vi "PLC.Dial800.OPC Read.vi"(6 "Timeout_ms":i32=500, 7 "Waif for Update":bool, 8 "error in (no error)":errorcluster, 9 "IncludeSN":bool=TRUE, 10 "Var URLs":T2[](array[typedef]), 11 "PLC Variables In":T1) -> (0 "error out":errorcluster, 1 "Duration(s)":dbl format="%.3f", 3 "PLC Variables":T1)   [LabVIEW 2018]
uses:
  PLC.Dial800.Var URL Item.ctl
  PLC.Dial800.VarNameSelector.ctl
  PLC.800 Variables.ctl
  <vilib>/KATE/Time/Time Utils.lvlib
panel:
  out "Durs":dbl[](array[numeric]) format="%.3f"
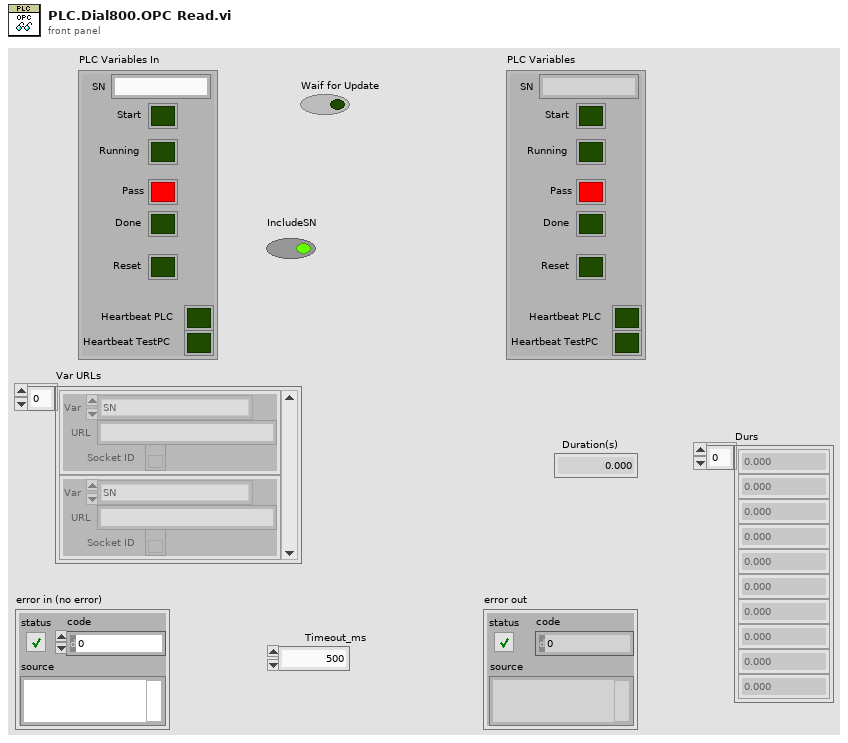
[diagram p1: front panel]
types:
  T1 = typedef "PLC.800 Variables.ctl" = cluster{"SN":string, "Start":bool, "Pass":bool, "Done":bool, "Running":bool, "Heartbeat PLC":bool, "Heartbeat TestPC":bool, "Reset":bool}
  T2 = typedef "PLC.Dial800.Var URL Item.ctl" = cluster{"Var":T3, "URL":string, "Socket ID":refnum<k13>}
  T3 = typedef "PLC.Dial800.VarNameSelector.ctl" = enum16{"SN", "Reset", "HeartBeat_PLC", "Heartbeat_PC", "Start", "Running", "Done", "Pass"}
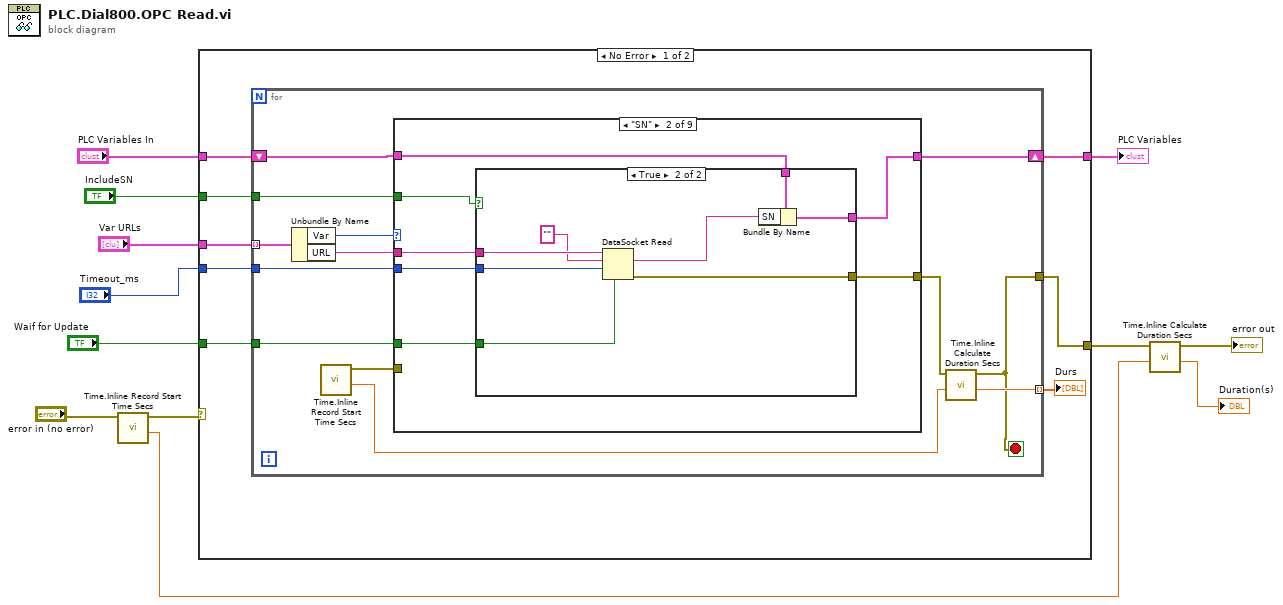
[diagram p0: block diagram]
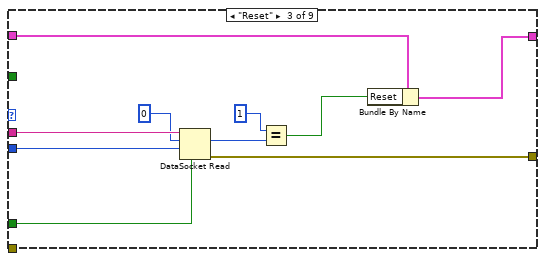
[diagram p4: hidden frame]
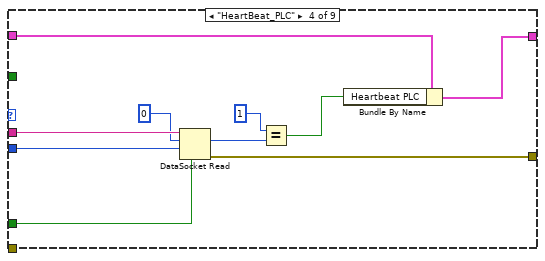
[diagram p5: hidden frame]
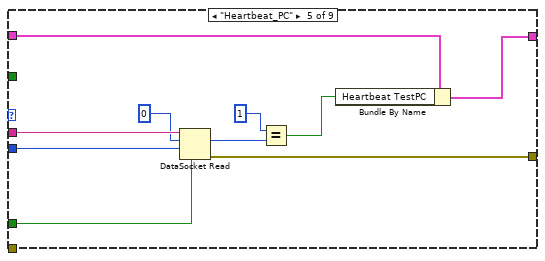
[diagram p6: hidden frame]
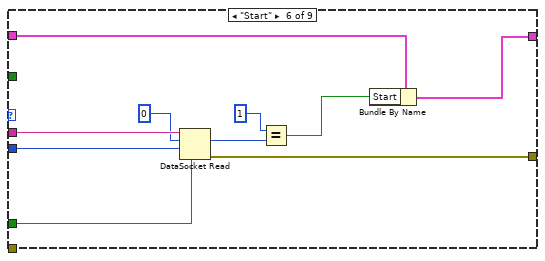
[diagram p7: hidden frame]
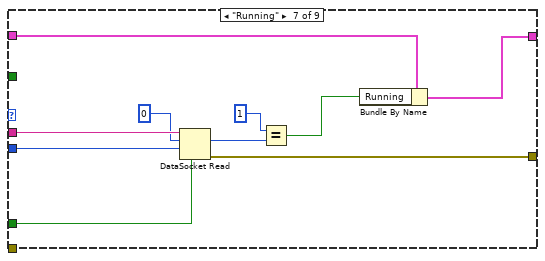
[diagram p8: hidden frame]
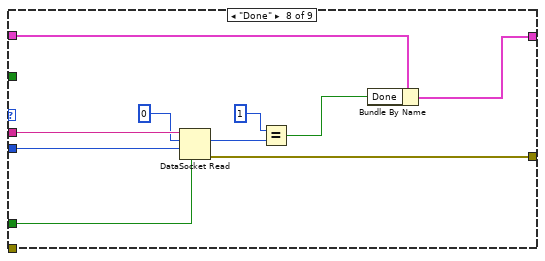
[diagram p9: hidden frame]
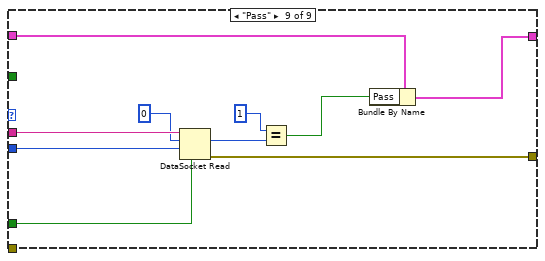
[diagram p10: hidden frame]
diagram:
  n1 = call <vilib>:"Time.Inline Record Start Time Secs.vi"("Error In Upper"="error in (no error)") -> ("Start(s)"=w4:dbl, "Error Out Upper"=w7:errorcluster)  [unwired: 8 in, 1 out]
  n2 = case shown="No Error" w7 {
    selector: w7 -> [_ w122]
    tunnel: [w16 w122] -> w6
    tunnel: "Var URLs" -> [w20 _]
    tunnel: "PLC Variables In" -> [w19 w121]
    tunnel: [w18 w121] -> w10
    tunnel: "Timeout_ms" -> [w17 _]
    tunnel: "Waif for Update" -> [w15 _]
    tunnel: "IncludeSN" -> [w13 _]
    frame No Error {
      n3 = for {
        tunnel: w20 -> [w33] mode=indexing
        shift-right: [w30] -> w18
        shift-left: w19 -> [w31]
        tunnel: w17 -> [w28]
        tunnel: [w22] -> w16
        tunnel: w15 -> [w27]
        tunnel: [w24] -> w14 mode=indexing
        tunnel: w13 -> [w23]
        stop <- w22 stop-if-true
        n4 = Unbundle By Name(w33) -> ("Var"=w32:T3, "URL"=w29:string)
        n5 = call <vilib>:"Time.Inline Record Start Time Secs.vi"() -> ("Start(s)"=w26:dbl, "Error Out Upper"=w25:errorcluster)  [unwired: 9 in, 1 out]
        n6 = case shown="\"SN\"" w32 {
          tunnel: w31 -> [w34 w41 w60 w70 w80 w90 w100 w110 w120]
          tunnel: [w34 w40 w59 w69 w79 w89 w99 w109 w119] -> w30
          tunnel: w29 -> [_ w39 w58 w68 w78 w88 w98 w108 w118]
          tunnel: w28 -> [_ w38 w57 w67 w77 w87 w97 w107 w117]
          tunnel: [_ w37 w56 w66 w76 w86 w96 w106 w116] -> w21
          tunnel: w27 -> [_ w36 w51 w61 w71 w81 w91 w101 w111]
          tunnel: w25 -> [_ _ _ _ _ _ _ _ _]
          tunnel: w23 -> [_ w35 _ _ _ _ _ _ _]
          frame Default {
          }
          frame "SN" {
            n7 = case shown="True" w35 {
              tunnel: w41 -> [w42 w50]
              tunnel: [w42 w49] -> w40
              tunnel: w39 -> [_ w48]
              tunnel: w38 -> [_ w45]
              tunnel: [_ w44] -> w37
              tunnel: w36 -> [_ w43]
              frame False {
              }
              frame True {
                n8 = DataSocket Read(6:w43, 9:w45, 10:"", 11:w48) -> (0:w44:errorcluster, 2:w46:string)  [unwired: 1 in, 5 out]
                n9 = Bundle By Name(cluster=w50, "SN"=w46) -> (w49:T1)
              }
            }
          }
          frame "Reset" {
            n10 = DataSocket Read(6:w51, 9:w57, 10:0, 11:w58) -> (0:w56:errorcluster, 2:w54:i32)  [unwired: 1 in, 5 out]
            n11 = Equal?(x=1, y=w54) -> (x = y?=w52:bool)
            n12 = Bundle By Name(cluster=w60, "Reset"=w52) -> (w59:T1)
          }
          frame "HeartBeat_PLC" {
            n13 = DataSocket Read(6:w61, 9:w67, 10:0, 11:w68) -> (0:w66:errorcluster, 2:w64:i32)  [unwired: 1 in, 5 out]
            n14 = Equal?(x=1, y=w64) -> (x = y?=w62:bool)
            n15 = Bundle By Name(cluster=w70, "Heartbeat PLC"=w62) -> (w69:T1)
          }
          frame "Heartbeat_PC" {
            n16 = DataSocket Read(6:w71, 9:w77, 10:0, 11:w78) -> (0:w76:errorcluster, 2:w74:i32)  [unwired: 1 in, 5 out]
            n17 = Equal?(x=1, y=w74) -> (x = y?=w72:bool)
            n18 = Bundle By Name(cluster=w80, "Heartbeat TestPC"=w72) -> (w79:T1)
          }
          frame "Start" {
            n19 = DataSocket Read(6:w81, 9:w87, 10:0, 11:w88) -> (0:w86:errorcluster, 2:w84:i32)  [unwired: 1 in, 5 out]
            n20 = Equal?(x=1, y=w84) -> (x = y?=w82:bool)
            n21 = Bundle By Name(cluster=w90, "Start"=w82) -> (w89:T1)
          }
          frame "Running" {
            n22 = DataSocket Read(6:w91, 9:w97, 10:0, 11:w98) -> (0:w96:errorcluster, 2:w94:i32)  [unwired: 1 in, 5 out]
            n23 = Equal?(x=1, y=w94) -> (x = y?=w92:bool)
            n24 = Bundle By Name(cluster=w100, "Running"=w92) -> (w99:T1)
          }
          frame "Done" {
            n25 = DataSocket Read(6:w101, 9:w107, 10:0, 11:w108) -> (0:w106:errorcluster, 2:w104:i32)  [unwired: 1 in, 5 out]
            n26 = Equal?(x=1, y=w104) -> (x = y?=w102:bool)
            n27 = Bundle By Name(cluster=w110, "Done"=w102) -> (w109:T1)
          }
          frame "Pass" {
            n28 = DataSocket Read(6:w111, 9:w117, 10:0, 11:w118) -> (0:w116:errorcluster, 2:w114:i32)  [unwired: 1 in, 5 out]
            n29 = Equal?(x=1, y=w114) -> (x = y?=w112:bool)
            n30 = Bundle By Name(cluster=w120, "Pass"=w112) -> (w119:T1)
          }
        }
        n31 = call <vilib>:"Time.Inline Calculate Duration Secs.vi"("Start(Sec)"=w26, "Error In Top"=w21) -> ("Duration(s)"=w24:dbl, "Error Out Top"=w22:errorcluster)  [unwired: 7 in, 1 out]
      }
      "Durs" <- w14
    }
    frame Error {
    }
  }
  "PLC Variables" <- w10
  n32 = call <vilib>:"Time.Inline Calculate Duration Secs.vi"("Start(Sec)"=w4, "Error In Top"=w6) -> ("Duration(s)"=→"Duration(s)":dbl, "Error Out Top"=→"error out":errorcluster)  [unwired: 7 in, 1 out]
